vi "Main.vi"() -> ()   [LabVIEW 2012]
panel:
  out "x+1":dbl
  in  "stop":bool
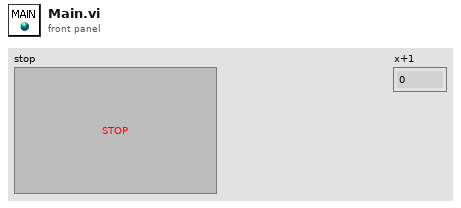
[diagram p1: front panel]
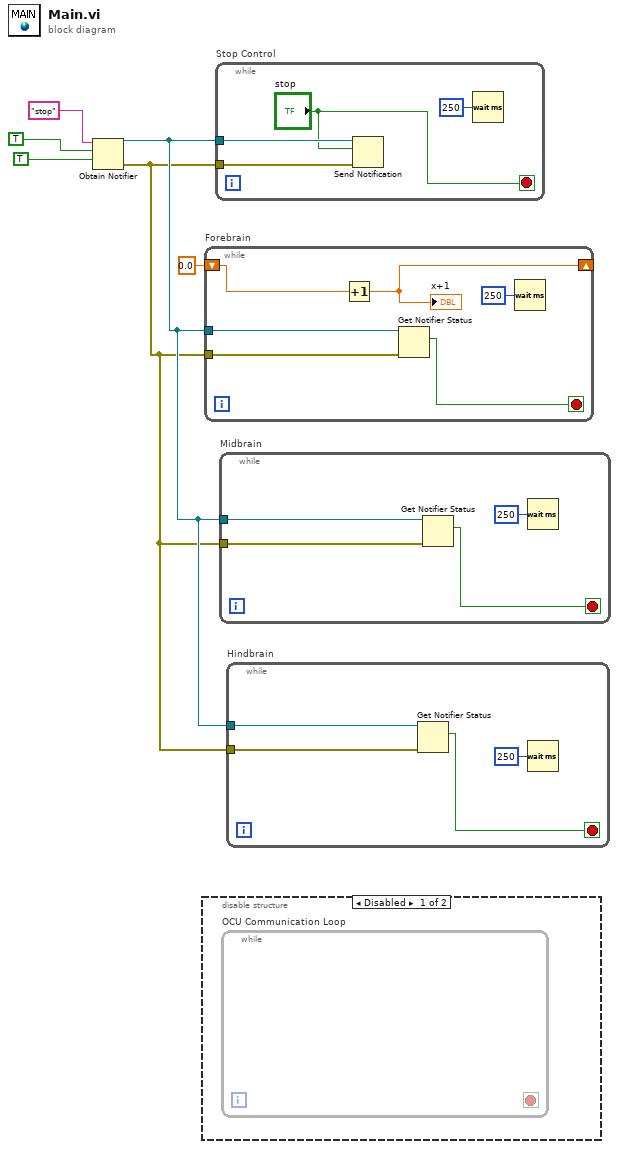
[diagram p0: block diagram]
diagram:
  n1 = Obtain Notifier(name (unnamed)="stop", notification data type=TRUE ("create if not found? (T)"), create if not found? (T)=TRUE) -> (notifier out=w3:refnum<notifier>, error out=w2:errorcluster)  [unwired: 1 in, 1 out]
  n2 = disable-structure shown="Disabled" {
    frame Disabled {
      n3 = while "OCU Communication Loop" {
        stop <- _ stop-if-true
      }
    }
    frame Enabled {
    }
  }
  n4 = while "Forebrain" {
    tunnel: w3 -> [w12]
    tunnel: w2 -> [w11]
    shift-right: [w8] -> _
    shift-left: 0.0 -> [w7]
    stop <- w10 stop-if-true
    n5 = Increment(x=w7) -> (x+1=w8:dbl)
    "x+1" <- w8
    n6 = Get Notifier Status(notifier=w12, error in (no error)=w11) -> (current notification=w10:bool)  [unwired: 4 out]
    n7 = Wait (ms)(milliseconds to wait=u32 250) -> ()  [unwired: 1 out]
  }
  n8 = while "Stop Control" {
    tunnel: w2 -> [w16]
    tunnel: w3 -> [w15]
    stop <- "stop" stop-if-true
    n9 = Send Notification(notification="stop", notifier=w15, error in (no error)=w16) -> ()  [unwired: 2 out]
    n10 = Wait (ms)(milliseconds to wait=u32 250) -> ()  [unwired: 1 out]
  }
  n11 = while "Midbrain" {
    tunnel: w3 -> [w19]
    tunnel: w2 -> [w18]
    stop <- w20 stop-if-true
    n12 = Get Notifier Status(notifier=w19, error in (no error)=w18) -> (current notification=w20:bool)  [unwired: 4 out]
    n13 = Wait (ms)(milliseconds to wait=u32 250) -> ()  [unwired: 1 out]
  }
  n14 = while "Hindbrain" {
    tunnel: w3 -> [w24]
    tunnel: w2 -> [w23]
    stop <- w22 stop-if-true
    n15 = Get Notifier Status(notifier=w24, error in (no error)=w23) -> (current notification=w22:bool)  [unwired: 4 out]
    n16 = Wait (ms)(milliseconds to wait=u32 250) -> ()  [unwired: 1 out]
  }
